vi "fotoncounter+lockin+fastratio_LV2010 GF VARIANT.vi"() -> ()   [LabVIEW 2014]
uses:
  Instance          14 40Saved   fotoncounter+lockin+fastratio v1 .vi
  Instance          13 40Saved   fotoncounter+lockin+fastratio v1 .vi
  Instance          33 40Saved   fotoncounter+lockin+fastratio v1 .vi
  Instance           2 40Saved   fotoncounter+lockin+fastratio v1 .vi
  Instance           5 40Saved   fotoncounter+lockin+fastratio v1 .vi
  Instance           6 40Saved   fotoncounter+lockin+fastratio v1 .vi
  Instance           7 40Saved   fotoncounter+lockin+fastratio v1 .vi
  Instance          15 40Saved   fotoncounter+lockin+fastratio v1 .vi
  Instance           8 40Saved   fotoncounter+lockin+fastratio v1 .vi
  Instance           9 40Saved   fotoncounter+lockin+fastratio v1 .vi
  Instance          10 40Saved   fotoncounter+lockin+fastratio v1 .vi
  Instance          11 40Saved   fotoncounter+lockin+fastratio v1 .vi
  Instance           1 40Saved   fotoncounter+lockin+fastratio v1 .vi
  Instance          18 40Saved   fotoncounter+lockin+fastratio v1 .vi
  Instance          19 40Saved   fotoncounter+lockin+fastratio v1 .vi
  Instance          23 40Saved   fotoncounter+lockin+fastratio v1 .vi
  Instance          17 40Saved   fotoncounter+lockin+fastratio v1 .vi
  Instance          22 40Saved   fotoncounter+lockin+fastratio v1 .vi
  Instance          20 40Saved   fotoncounter+lockin+fastratio v1 .vi
  Instance          21 40Saved   fotoncounter+lockin+fastratio v1 .vi
  Instance          26 40Saved   fotoncounter+lockin+fastratio v1 .vi
  Instance          27 40Saved   fotoncounter+lockin+fastratio v1 .vi
  Instance          29 40Saved   fotoncounter+lockin+fastratio v1 .vi
  <vilib>/Utility/file.llb/Write To Spreadsheet File (DBL).vi
  Instance          24 40Saved   fotoncounter+lockin+fastratio v1 .vi
  <vilib>/Utility/file.llb/Read From Spreadsheet File (DBL).vi
  Instance          32 40Saved   fotoncounter+lockin+fastratio v1 .vi
  Instance          31 40Saved   fotoncounter+lockin+fastratio v1 .vi
  Instance          30 40Saved   fotoncounter+lockin+fastratio v1 .vi
panel:
  in  "error in (no error)":errorcluster
  out "error out":errorcluster
  in  "Cluster":T1={"slope"=1, "Input Mode"=0, "time constant"=0, "display type"=0, "Range"=6} {"Range" items=["100 nV", "300 nV", "1 uV", "3 uV", "10 uV", "30 uV", "100 uV", "300 uV", "1 mV", "3 mV", "10 mV", "30 mV", "100 mV", "300 mV", "1 V", "3 V"]; "display type" items=["Output %", "Output calibrated ", "Ratio", "log Ratio", "ADC 1", "ADC 2", " ADC 3", "ADC 4", "Noise %", "Noise Calibrated", "Ref. Frequency"]; "time constant" items=["1 ms", "3 ms", "10 ms", "30 ms", "100 ms", "300 ms", "1 s", "3 s", "10 s", "30 s", "100 s", "300 s", "1 ks", "3 ks"]; "Input Mode" items=["Voltage Input ( A or A-B)", "Current Input 10E6 V/A", "Current Input 10E8 V/A"]; "slope" items=["6dB/octave", "12dB/octave"]}
  out "lockin":i32
  out "counter B":i32=147
  out "counter A":i32=5821
  out "LOCKIN OUTPUT DATA":cluster{"Y":dbl[], "Y":dbl[]}[](graph)=[{"Y"=[1.0], "Y"=[0.08234234]}]
  in  "EG&G 5209\nlockin amplifier\nGPIB address":u8=12 min=1 max=32 step=1
  out "# count periods done":i32=1
  out "Data Bit value":i32=1
  out "PHOTON COUNTER DATA":cluster{"all rows":dbl[], "all rows":dbl[]}[](graph)=[{"all rows"=[1.0], "all rows"=[5821.0]}, {"all rows"=[1.0], "all rows"=[147.0]}]
  in  "T select":i16(slide) scale=0.0..2.0
  in  "A scan step (V)":ext=-0.005 format="%.3e"
  in  "B scan step(V)":ext=-0.005 format="%.3e"
  in  "T scan step (V)":ext=0.02 format="%.3e"
  out "error 7":bool
  in  "A mode":bool=TRUE
  in  "B mode":bool=TRUE
  in  "T mode":bool=TRUE
  in  "A level (V)":ext=-0.025 format="%.3e"
  in  "B level (V)":ext=-0.025 format="%.3e"
  in  "T level (V)":ext=-0.01 format="%.3e"
  in  "B Preset":ext=1.0
  in  "count mode":i16(slide) scale=0.0..3.0 scale format="%.2f"
  in  "Path":path=path "C:/lvtemp/phototemp"
  out "error 6":bool
  in  "A slope":bool
  in  "B slope":bool
  in  "T slope":bool
  in  "trigger slope":bool
  out "error 5":bool
  in  "trigger level":ext=2.0 format="%.3f"
  in  "A scan step":ext=0.000005 format="%.3e"
  in  "dwell source":i32(slide) scale=0.0..1.0
  in  "dwell time":ext=0.1 format="%.4f"
  in  "# count periods\n(2000 max.)":i32=1
  in  "A select":i16(slide)=1 scale=0.0..1.0
  in  "B select":i16(slide)=1 scale=1.0..2.0 scale format="%.2f"
  in  "SR400\nphoton counter\nGPIB address":string="0:23"
  in  "B gate delay":ext=0.00027000000000000000001 format="%.3e"
  in  "B gate mode":i16(slide)=1 scale=0.0..2.0
  out "error 2":bool
  in  "B gate width":ext=0.00021 format="%.3e"
  in  "B scan step":ext=0.000005 format="%.3e"
  in  "A gate delay":ext=0.00001 format="%.3e"
  in  "A gate mode":i16(slide)=1 scale=0.0..2.0 scale format="%.2f"
  in  "A gate width":ext=0.00021 format="%.3e"
  in  "T Preset":ext=1.0
  # "SR400 PHOTON COUNTER + EG&G 5209 LOCKIN AMPLIFIER"
  # "ADDRESSING/TRIGGER/DWELL SETTINGS"
  # "COUNTER/INPUT SETTINGS"
  # "photon counter GPIB Board 0, address 23\nEG&G lockin GPIB Board 0, address 12"
  # "RISE\n\nFALL"
  # "(s)"
  # "note: valid dwell time\n0.002  to 60.0 s"
  # "(s)"
  # "DISCRIMINATOR SETTINGS"
  # "GATE SETTINGS"
  # "FIXED\n\nSCAN"
  # "RISE\n\nFALL"
  # "RISE\n\nFALL"
  # "FIXED\n\nSCAN"
  # "FIXED\n\nSCAN"
  # "RISE\n\nFALL"
  # "note: valid disc levels \n-0.30 to 0.30 V"
  # "note: valid scan steps \n-0.020 to 0.020 V"
  # "\"...The greatest trick the Devil ever pulled was convincing the world he didn't exist...\" (and then inventing LabView)..."
  # "This makes the lockin work again. no idea if the settings are right, or even need to be messed with"
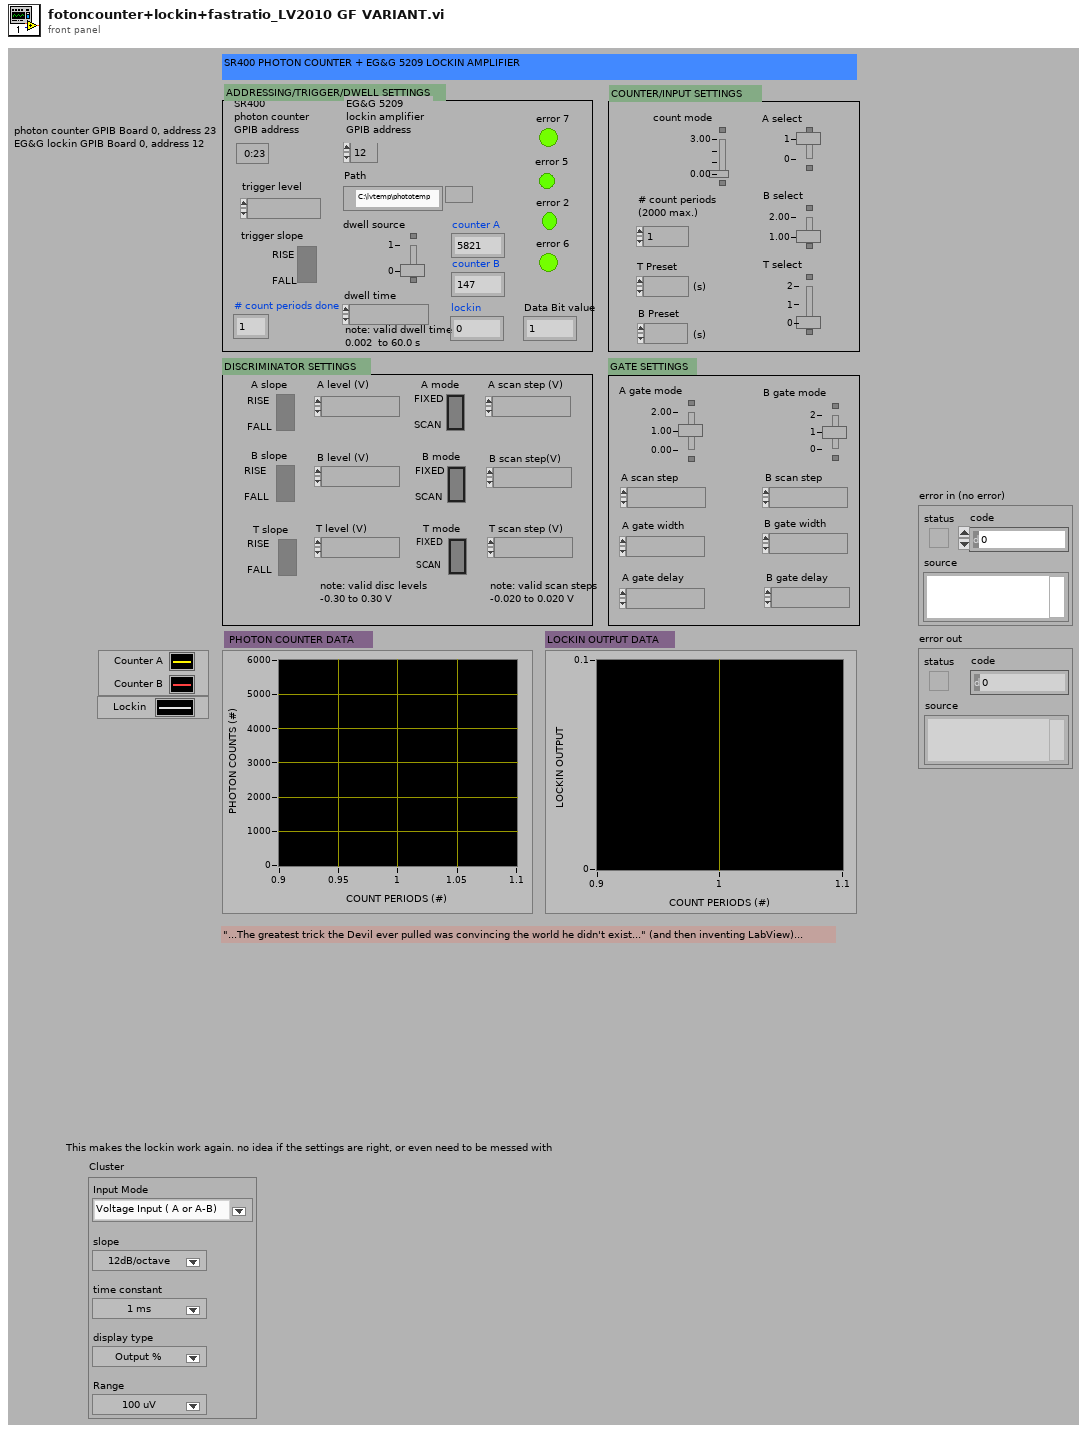
[diagram p1: front panel]
types:
  T1 = cluster{"slope":i32, "Input Mode":i32, "time constant":i32, "display type":i32, "Range":i32}
  T2 = enum16{"open", "open or create", "create or replace", "create", "open (read only)"}
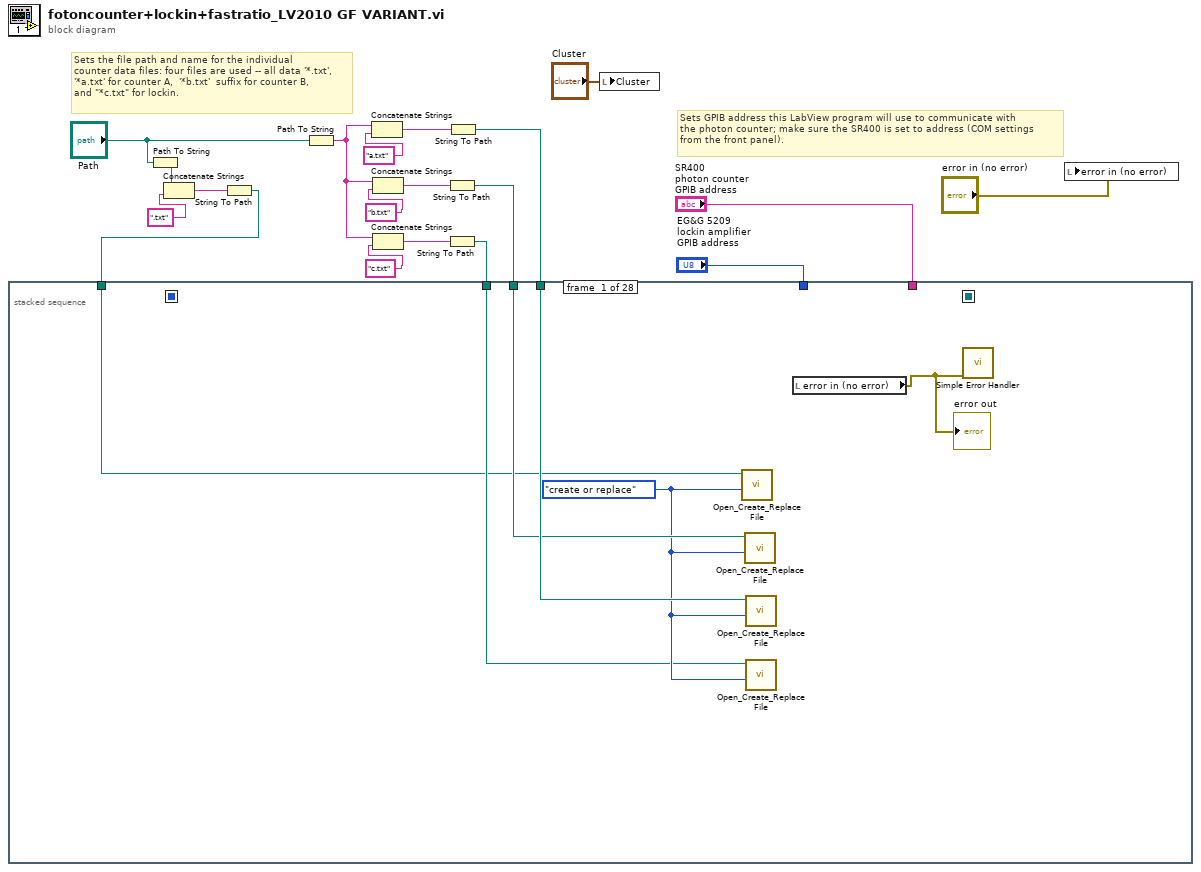
[diagram p0: block diagram]
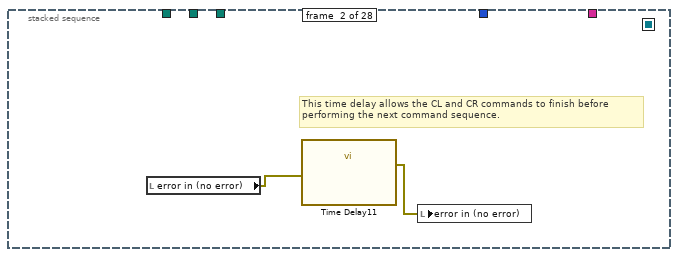
[diagram p2: hidden frame]
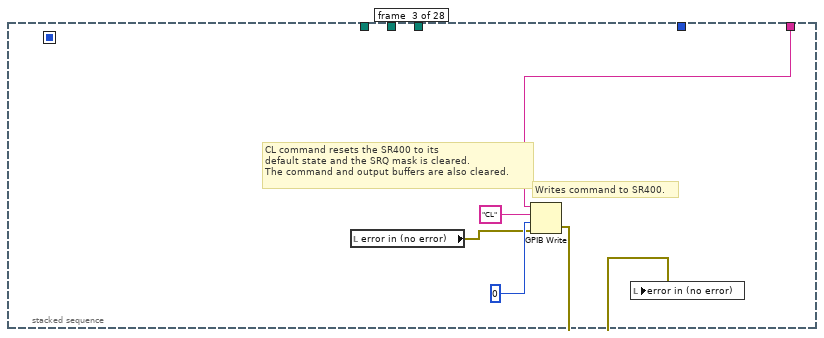
[diagram p3: hidden frame]
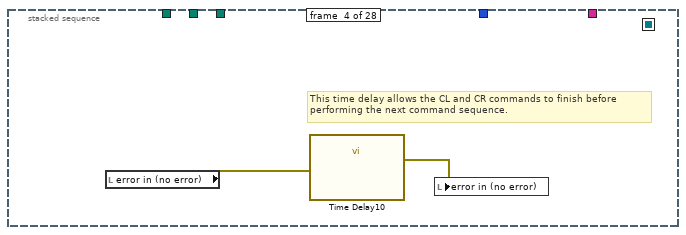
[diagram p4: hidden frame]
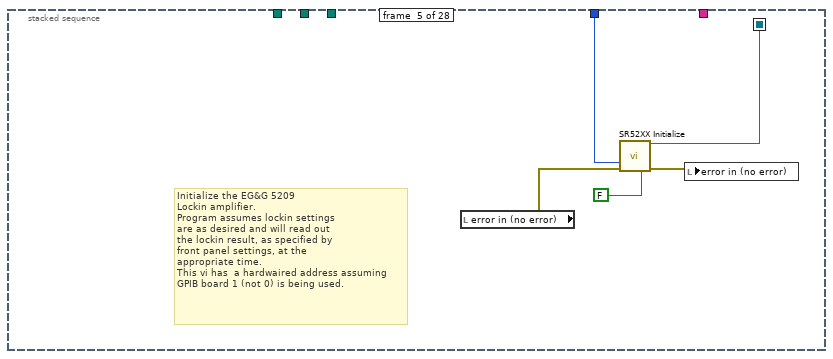
[diagram p5: hidden frame]
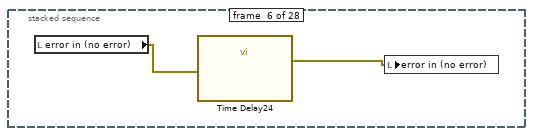
[diagram p6: hidden frame]
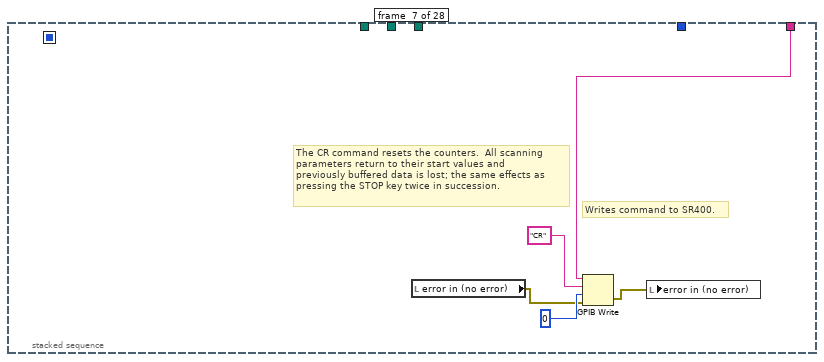
[diagram p7: hidden frame]
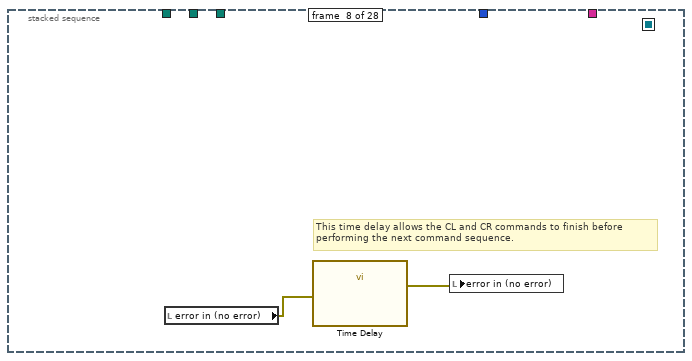
[diagram p8: hidden frame]
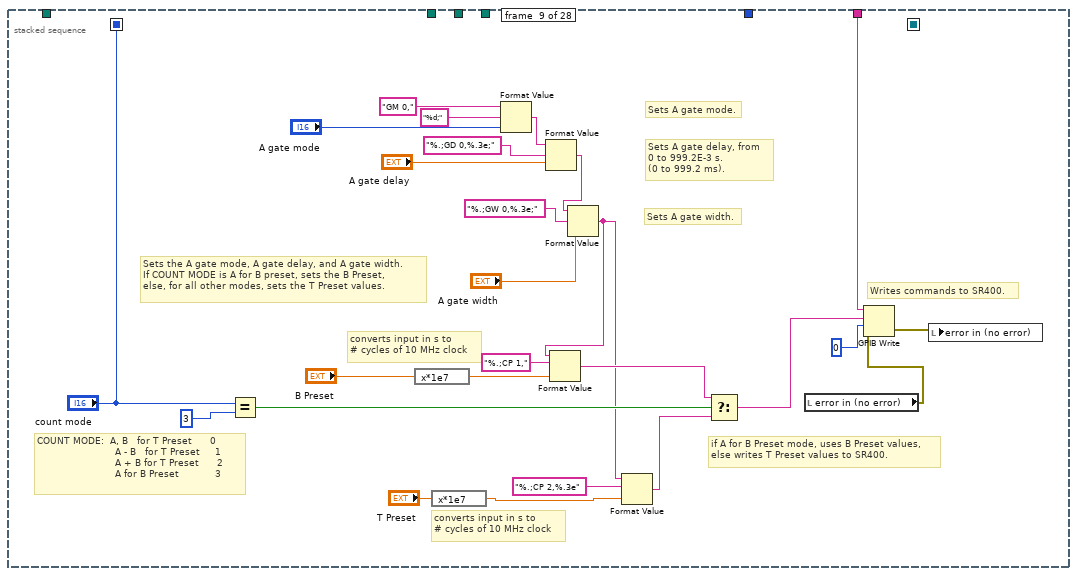
[diagram p9: hidden frame]
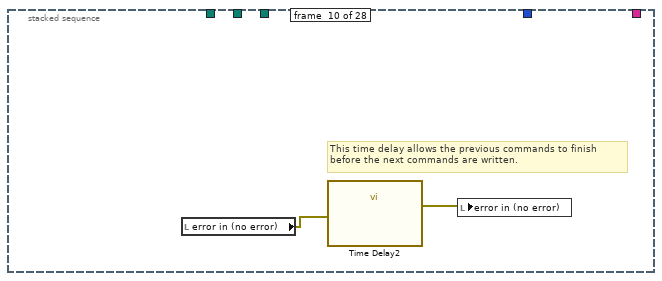
[diagram p10: hidden frame]
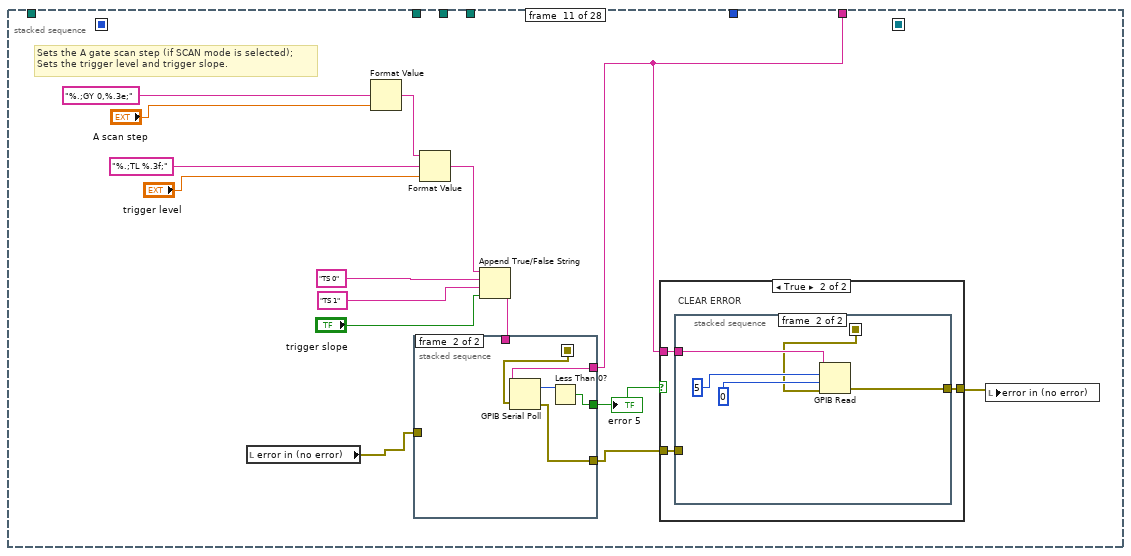
[diagram p11: hidden frame]
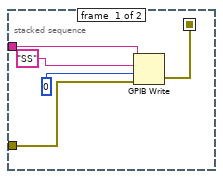
[diagram p13: hidden frame]
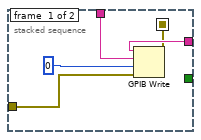
[diagram p14: hidden frame]
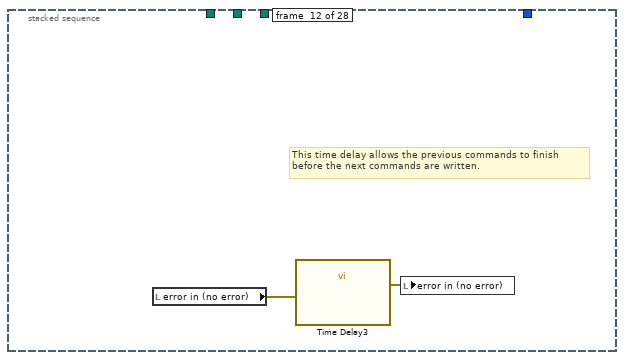
[diagram p15: hidden frame]
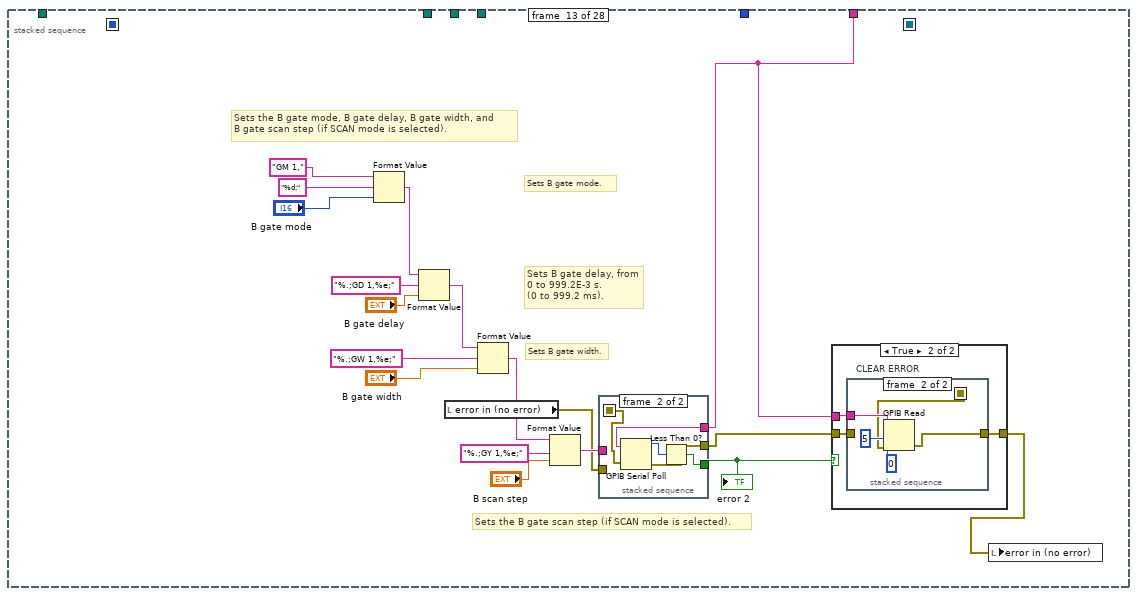
[diagram p16: hidden frame]
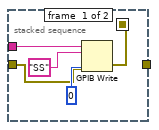
[diagram p18: hidden frame]
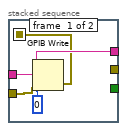
[diagram p19: hidden frame]
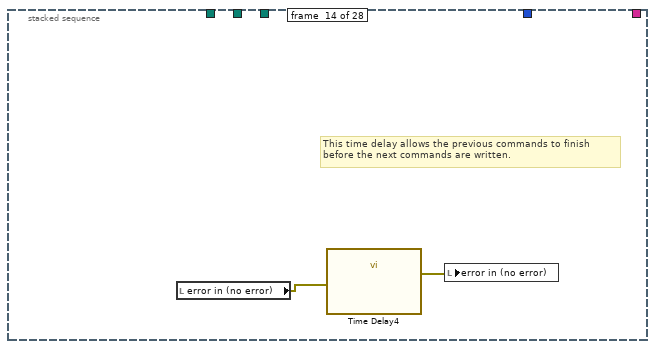
[diagram p20: hidden frame]
diagram:
  # "Sets the file path and name for the individual\ncounter data files: four files are used -- all data '*.txt',\n'*a.txt' for counter A,  '*b.txt'  suffix for counter B,\nand \"*c.txt\" for lockin."
  # "Sets GPIB address this LabView program will use to communicate with\nthe photon counter; make sure the SR400 is set to address (COM settings\nfrom the front panel)."
  n1 = Path To String(path="Path") -> (string=w13:string)
  n2 = Concatenate Strings(w13, ".txt") -> (w11:string)
  n3 = String To Path(string=w11) -> (path=w3:path)
  n4 = Path To String(path="Path") -> (string=w6:string)
  n5 = Concatenate Strings(w6, "a.txt") -> (w14:string)
  n6 = Concatenate Strings(w6, "b.txt") -> (w17:string)
  n7 = Concatenate Strings(w6, "c.txt") -> (w8:string)
  n8 = String To Path(string=w17) -> (path=w15:path)
  n9 = String To Path(string=w8) -> (path=w5:path)
  n10 = String To Path(string=w14) -> (path=w16:path)
  n11 = stacked-sequence {
    seq-local: [_ _ _ _ _ _ _ _ "count mode" _ _ _ _ _ _ _ _ _ _ _ _ _ _ _ _ _ _ _] -> [_ _ _ _ _ _ _ _ _ _ _ _ _ _ _ _ _ _ _ _ _ _ _ _ _ _ w274 _]
    seq-local: [_ _ _ _ w37 _ _ _ _ _ _ _ _ _ _ _ _ _ _ _ _ _ _ _ _ _ _ _] -> [_ _ _ _ _ _ _ _ _ _ _ _ _ _ _ _ _ _ _ _ _ _ _ _ _ _ w273 _]
    tunnel: "SR400\nphoton counter\nGPIB address" -> [_ _ w30 _ _ _ w44 _ w69 _ w80 _ w122 _ w166 _ w179 _ w189 _ w203 _ w231 _ w259 _ w280 _]
    tunnel: w16 -> [w25 _ _ _ _ _ _ _ _ _ _ _ _ _ _ _ _ _ _ _ _ _ _ _ _ _ w279 _]
    tunnel: w15 -> [w24 _ _ _ _ _ _ _ _ _ _ _ _ _ _ _ _ _ _ _ _ _ _ _ _ _ w278 _]
    tunnel: w3 -> [w21 _ _ _ _ _ _ _ _ _ _ _ _ _ _ _ _ _ _ _ _ _ _ _ _ _ w277 w469]
    tunnel: "EG&G 5209\nlockin amplifier\nGPIB address" -> [_ _ _ _ w38 _ _ _ _ _ _ _ _ _ _ _ _ _ _ _ _ _ _ _ _ _ _ _]
    tunnel: w5 -> [w22 _ _ _ _ _ _ _ _ _ _ _ _ _ _ _ _ _ _ _ _ _ _ _ _ _ w276 _]
    frame #0 {
      w23 = T2."create or replace" ("function (open:0)")
      n12 = call <vilib>:"Open_Create_Replace File.vi"("function (open:0)"=w23, "file path"=w21) -> ()  [unwired: 6 in, 4 out]
      n13 = call <vilib>:"Open_Create_Replace File.vi"("function (open:0)"=w23, "file path"=w24) -> ()  [unwired: 6 in, 4 out]
      n14 = call <vilib>:"Open_Create_Replace File.vi"("function (open:0)"=w23, "file path"=w25) -> ()  [unwired: 6 in, 4 out]
      n15 = call <vilib>:"Open_Create_Replace File.vi"("function (open:0)"=w23, "file path"=w22) -> ()  [unwired: 6 in, 4 out]
      n16 = local read "error in (no error)"() -> (w20:errorcluster)
      "error out" <- w20
      n17 = call <vilib>:"Simple Error Handler.vi"("error in (no error)"=w20) -> ()  [unwired: 4 in, 5 out]
    }
    frame #1 {
      # "This time delay allows the CL and CR commands to finish before\nperforming the next command sequence."
      n18 = local read "error in (no error)"() -> (w27:errorcluster)
      n19 = call "Time Delay11"("error in (no error)"=w27) -> ("error out"=w26:errorcluster)  [unwired: 10 in]
      n20 = local write "error in (no error)"(w26) -> ()
    }
    frame #2 {
      # "Writes command to SR400."
      # "CL command resets the SR400 to its\ndefault state and the SRQ mask is cleared.\nThe command and output buffers are also cleared."
      n21 = local read "error in (no error)"() -> (w29:errorcluster)
      n22 = GPIB Write(0:w30, 1:"CL", 2:0, 3:w29) -> (6:w28:errorcluster)  [unwired: 1 in, 1 out]
      n23 = local write "error in (no error)"(w28) -> ()
    }
    frame #3 {
      # "This time delay allows the CL and CR commands to finish before\nperforming the next command sequence."
      n24 = local read "error in (no error)"() -> (w33:errorcluster)
      n25 = call "Time Delay10"("error in (no error)"=w33) -> ("error out"=w34:errorcluster)  [unwired: 10 in]
      n26 = local write "error in (no error)"(w34) -> ()
    }
    frame #4 {
      # "Initialize the EG&G 5209\nLockin amplifier.\nProgram assumes lockin settings\nare as desired and will read out\nthe lockin result, as specified by \nfront panel settings, at the\nappropriate time.\nThis vi has  a hardwaired address assuming \nGPIB board 1 (not 0) is being used."
      n27 = local read "error in (no error)"() -> (w35:errorcluster)
      n28 = call "SR52XX Initialize.vi"("Port"=w38, "error in (no error)"=w35, "reset"=FALSE) -> ("VISA session"=w37:refnum<visa-resource-name>, "error out"=w36:errorcluster)  [unwired: 10 in, 1 out]
      n29 = local write "error in (no error)"(w36) -> ()
    }
    frame #5 {
      n30 = local read "error in (no error)"() -> (w40:errorcluster)
      n31 = call "Time Delay24"("error in (no error)"=w40) -> ("error out"=w41:errorcluster)  [unwired: 10 in]
      n32 = local write "error in (no error)"(w41) -> ()
    }
    frame #6 {
      # "Writes command to SR400."
      # "The CR command resets the counters.  All scanning\nparameters return to their start values and \npreviously buffered data is lost; the same effects as\npressing the STOP key twice in succession."
      n33 = local read "error in (no error)"() -> (w42:errorcluster)
      n34 = GPIB Write(0:w44, 1:"CR", 2:0, 3:w42) -> (6:w43:errorcluster)  [unwired: 1 in, 1 out]
      n35 = local write "error in (no error)"(w43) -> ()
    }
    frame #7 {
      # "This time delay allows the CL and CR commands to finish before\nperforming the next command sequence."
      n36 = local read "error in (no error)"() -> (w48:errorcluster)
      n37 = call "Time Delay"("error in (no error)"=w48) -> ("error out"=w47:errorcluster)  [unwired: 10 in]
      n38 = local write "error in (no error)"(w47) -> ()
    }
    frame #8 {
      # "if A for B Preset mode, uses B Preset values,\nelse writes T Preset values to SR400."
      # "converts input in s to\n# cycles of 10 MHz clock"
      # "converts input in s to\n# cycles of 10 MHz clock"
      # "Writes commands to SR400."
      # "Sets A gate delay, from \n0 to 999.2E-3 s.\n(0 to 999.2 ms)."
      # "Sets A gate width."
      # "Sets A gate mode."
      # "COUNT MODE:  A, B   for T Preset      0 \n                          A - B   for T Preset     1\n                          A + B for T Preset      2\n                          A for B Preset            3"
      # "Sets the A gate mode, A gate delay, and A gate width.\nIf COUNT MODE is A for B preset, sets the B Preset, \nelse, for all other modes, sets the T Preset values."
      n39 = Equal?(x="count mode", y=3) -> (x = y?=w61:bool)
      n40 = expression code="x*1e7"("B Preset") -> (w51:ext)
      n41 = expression code="x*1e7"("T Preset") -> (w53:ext)
      n42 = Format Value(string ("")="GM 0,", format string="%d;", value (0)="A gate mode") -> (output string=w68:string)
      n43 = Format Value(string ("")=w68, format string="%.;GD 0,%.3e;", value (0)="A gate delay") -> (output string=w65:string)
      n44 = Format Value(string ("")=w65, format string="%.;GW 0,%.3e;", value (0)="A gate width") -> (output string=w56:string)
      n45 = Format Value(string ("")=w56, format string="%.;CP 1,", value (0)=w51) -> (output string=w57:string)
      n46 = Format Value(string ("")=w56, format string="%.;CP 2,%.3e", value (0)=w53) -> (output string=w59:string)
      n47 = Select(t=w57, s=w61, f=w59) -> (s? t:f=w55:string)
      n48 = local read "error in (no error)"() -> (w49:errorcluster)
      n49 = GPIB Write(0:w69, 1:w55, 2:0, 3:w49) -> (6:w50:errorcluster)  [unwired: 1 in, 1 out]
      n50 = local write "error in (no error)"(w50) -> ()
    }
    frame #9 {
      # "This time delay allows the previous commands to finish \nbefore the next commands are written."
      n51 = local read "error in (no error)"() -> (w76:errorcluster)
      n52 = call "Time Delay2"("error in (no error)"=w76) -> ("error out"=w75:errorcluster)  [unwired: 10 in]
      n53 = local write "error in (no error)"(w75) -> ()
    }
    frame #10 {
      # "Sets the A gate scan step (if SCAN mode is selected); \nSets the trigger level and trigger slope."
      n54 = local read "error in (no error)"() -> (w79:errorcluster)
      n55 = Format Value(format string="%.;GY 0,%.3e;", value (0)="A scan step") -> (output string=w84:string)  [unwired: 1 in]
      n56 = Format Value(string ("")=w84, format string="%.;TL %.3f;", value (0)="trigger level") -> (output string=w87:string)
      n57 = Append True/False String(1:"trigger slope", 2:"TS 1", 3:"TS 0", 4:w87) -> (0:w91:string)
      n58 = stacked-sequence {
        seq-local: [w106 _] -> [_ w112]
        tunnel: w80 -> [w109 w113]
        tunnel: w91 -> [w108 _]
        tunnel: [_ w115] -> w82
        tunnel: w79 -> [w107 _]
        tunnel: [_ w111] -> w78
        frame #0 {
          n59 = GPIB Write(0:w109, 1:w108, 2:0, 3:w107) -> (6:w106:errorcluster)  [unwired: 1 in, 1 out]
        }
        frame #1 {
          n60 = GPIB Serial Poll(0:w113, 1:w112) -> (2:w114:i16, 4:w111:errorcluster)  [unwired: 1 out]
          n61 = Less Than 0?(x=w114) -> (x < 0?=w115:bool)
        }
      }
      "error 5" <- w82
      n62 = case shown="True" w82 {
        tunnel: w80 -> [_ w95]
        tunnel: w78 -> [w92 w94]
        tunnel: [w92 w93] -> w77
        frame False {
          # "NO ERROR."
        }
        frame True {
          # "CLEAR ERROR"
          n63 = stacked-sequence {
            seq-local: [w96 _] -> [_ w102]
            tunnel: w95 -> [w98 w103]
            tunnel: w94 -> [w97 _]
            tunnel: [_ w101] -> w93
            frame #0 {
              n64 = GPIB Write(0:w98, 1:"SS", 2:0, 3:w97) -> (6:w96:errorcluster)  [unwired: 1 in, 1 out]
            }
            frame #1 {
              n65 = GPIB Read(0:w103, 1:5, 2:0, 3:w102) -> (7:w101:errorcluster)  [unwired: 1 in, 2 out]
            }
          }
        }
      }
      n66 = local write "error in (no error)"(w77) -> ()
    }
    frame #11 {
      # "This time delay allows the previous commands to finish \nbefore the next commands are written."
      n67 = local read "error in (no error)"() -> (w117:errorcluster)
      n68 = call "Time Delay3"("error in (no error)"=w117) -> ("error out"=w116:errorcluster)  [unwired: 10 in]
      n69 = local write "error in (no error)"(w116) -> ()
    }
    frame #12 {
      # "Sets the B gate scan step (if SCAN mode is selected)."
      # "Sets B gate width."
      # "Sets B gate delay, from \n0 to 999.2E-3 s.\n(0 to 999.2 ms)."
      # "Sets B gate mode."
      # "Sets the B gate mode, B gate delay, B gate width, and \nB gate scan step (if SCAN mode is selected)."
      n70 = Format Value(string ("")="GM 1,", format string="%d;", value (0)="B gate mode") -> (output string=w127:string)
      n71 = Format Value(string ("")=w127, format string="%.;GD 1,%e;", value (0)="B gate delay") -> (output string=w121:string)
      n72 = local read "error in (no error)"() -> (w120:errorcluster)
      n73 = Format Value(string ("")=w121, format string="%.;GW 1,%e;", value (0)="B gate width") -> (output string=w131:string)
      n74 = Format Value(string ("")=w131, format string="%.;GY 1,%e;", value (0)="B scan step") -> (output string=w134:string)
      n75 = stacked-sequence {
        seq-local: [w150 _] -> [_ w156]
        tunnel: w122 -> [w152 w157]
        tunnel: [_ w159] -> w135
        tunnel: w134 -> [w154 _]
        tunnel: w120 -> [w151 _]
        tunnel: [_ w155] -> w119
        frame #0 {
          n76 = GPIB Write(0:w152, 1:w154, 2:0, 3:w151) -> (6:w150:errorcluster)  [unwired: 1 in, 1 out]
        }
        frame #1 {
          n77 = GPIB Serial Poll(0:w157, 1:w156) -> (2:w158:i16, 4:w155:errorcluster)  [unwired: 1 out]
          n78 = Less Than 0?(x=w158) -> (x < 0?=w159:bool)
        }
      }
      "error 2" <- w135
      n79 = case shown="True" w135 {
        tunnel: w122 -> [_ w139]
        tunnel: w119 -> [w136 w138]
        tunnel: [w136 w137] -> w118
        frame False {
          # "NO ERROR."
        }
        frame True {
          # "CLEAR ERROR"
          n80 = stacked-sequence {
            seq-local: [w140 _] -> [_ w146]
            tunnel: w139 -> [w142 w147]
            tunnel: w138 -> [w141 _]
            tunnel: [_ w145] -> w137
            frame #0 {
              n81 = GPIB Write(0:w142, 1:"SS", 2:0, 3:w141) -> (6:w140:errorcluster)  [unwired: 1 in, 1 out]
            }
            frame #1 {
              n82 = GPIB Read(0:w147, 1:5, 2:0, 3:w146) -> (7:w145:errorcluster)  [unwired: 1 in, 2 out]
            }
          }
        }
      }
      n83 = local write "error in (no error)"(w118) -> ()
    }
    frame #13 {
      # "This time delay allows the previous commands to finish \nbefore the next commands are written."
      n84 = local read "error in (no error)"() -> (w161:errorcluster)
      n85 = call "Time Delay4"("error in (no error)"=w161) -> ("error out"=w160:errorcluster)  [unwired: 10 in]
      n86 = local write "error in (no error)"(w160) -> ()
    }
    frame #14 {
      # "Writes commands to SR400."
      # "Sets the input to counter A (INPUT1 or 10 MHz clock);\nSets the input to counter B (INPUT1 or INPUT2);"
      n87 = Format Value(string ("")="CI 0,", format string="%d;", value (0)="A select") -> (output string=w171:string)
      n88 = Format Value(string ("")=w171, format string="%.;CI 1,%d;", value (0)="B select") -> (output string=w164:string)
      n89 = local read "error in (no error)"() -> (w163:errorcluster)
      n90 = GPIB Write(0:w166, 1:w164, 2:0, 3:w163) -> (6:w162:errorcluster)  [unwired: 1 in, 1 out]
      n91 = local write "error in (no error)"(w162) -> ()
    }
    frame #15 {
      # "This time delay allows the previous commands to finish \nbefore the next commands are written."
      n92 = local read "error in (no error)"() -> (w174:errorcluster)
      n93 = call "Time Delay12"("error in (no error)"=w174) -> ("error out"=w173:errorcluster)  [unwired: 10 in]
      n94 = local write "error in (no error)"(w173) -> ()
    }
    frame #16 {
      # "Writes commands to SR400."
      # "Sets the input to counter T (EXT TRIG, INPUT 2, or 10 MHz clock);"
      n95 = local read "error in (no error)"() -> (w176:errorcluster)
      n96 = Pick Line(string ("")="CI 2,", multi-line string="0;\r2;\r3;", line index="T select") -> (output string=w178:string)
      n97 = GPIB Write(0:w179, 1:w178, 2:0, 3:w176) -> (6:w175:errorcluster)  [unwired: 1 in, 1 out]
      n98 = local write "error in (no error)"(w175) -> ()
    }
    frame #17 {
      # "This time delay allows the previous commands to finish \nbefore the next commands are written."
      n99 = local read "error in (no error)"() -> (w184:errorcluster)
      n100 = call "Time Delay5"("error in (no error)"=w184) -> ("error out"=w183:errorcluster)  [unwired: 10 in]
      n101 = local write "error in (no error)"(w183) -> ()
    }
    frame #18 {
      # "Writes commands to SR400."
      # "B counter discriminator level"
      # "T counter discriminator level"
      # "A counter discriminator level"
      # "Sets the A, B, and T discriminator levels.  \nThe input values must be between \n-0.3 V and 0.3 V (-300 mV and 300 mV)\nor else the counter leaves the default values\nof -0.01 V (-10 mV)."
      n102 = Format Value(string ("")="DL 0,", format string="%.4e;DL 1,", value (0)="A level (V)") -> (output string=w193:string)
      n103 = Format Value(string ("")=w193, format string="%.4e;DL 2,", value (0)="B level (V)") -> (output string=w194:string)
      n104 = Format Value(string ("")=w194, format string="%.4e;", value (0)="T level (V)") -> (output string=w187:string)
      n105 = local read "error in (no error)"() -> (w186:errorcluster)
      n106 = GPIB Write(0:w189, 1:w187, 2:0, 3:w186) -> (6:w185:errorcluster)  [unwired: 1 in, 1 out]
      n107 = local write "error in (no error)"(w185) -> ()
    }
    frame #19 {
      # "This time delay allows the previous commands to finish \nbefore the next commands are written."
      n108 = local read "error in (no error)"() -> (w200:errorcluster)
      n109 = call "Time Delay7"("error in (no error)"=w200) -> ("error out"=w199:errorcluster)  [unwired: 10 in]
      n110 = local write "error in (no error)"(w199) -> ()
    }
    frame #20 {
      # "Sets the slope of the A, B, and T\ndiscriminator levels  (rise or fall)."
      n111 = local read "error in (no error)"() -> (w202:errorcluster)
      n112 = Append True/False String(1:"A slope", 2:"DS 0,1;", 3:"DS 0,0;") -> (0:w210:string)  [unwired: 1 in]
      n113 = Append True/False String(1:"B slope", 2:"DS 1,1;", 3:"DS 1,0;", 4:w210) -> (0:w213:string)
      n114 = Append True/False String(1:"T slope", 2:"DS 2,1;", 3:"DS 2,0;", 4:w213) -> (0:w216:string)
      n115 = stacked-sequence {
        seq-local: [w217 _] -> [_ w223]
        tunnel: w203 -> [w220 w226]
        tunnel: w216 -> [w221 _]
        tunnel: [_ w224] -> w206
        tunnel: w202 -> [w218 _]
        tunnel: [_ w222] -> w201
        frame #0 {
          n116 = GPIB Write(0:w220, 1:w221, 2:0, 3:w218) -> (6:w217:errorcluster)  [unwired: 1 in, 1 out]
        }
        frame #1 {
          n117 = GPIB Serial Poll(0:w226, 1:w223) -> (2:w225:i16, 4:w222:errorcluster)  [unwired: 1 out]
          n118 = Less Than 0?(x=w225) -> (x < 0?=w224:bool)
        }
      }
      "error 6" <- w206
      n119 = local write "error in (no error)"(w201) -> ()
    }
    frame #21 {
      # "This time delay allows the previous commands to finish \nbefore the next commands are written."
      n120 = local read "error in (no error)"() -> (w228:errorcluster)
      n121 = call "Time Delay8"("error in (no error)"=w228) -> ("error out"=w227:errorcluster)  [unwired: 10 in]
      n122 = local write "error in (no error)"(w227) -> ()
    }
    frame #22 {
      # "Sets the mode of the A, B, and T\ndiscriminators  (FIXED or SCAN)."
      n123 = local read "error in (no error)"() -> (w230:errorcluster)
      n124 = Append True/False String(1:"A mode", 2:"DM 0,1;", 3:"DM 0,0;") -> (0:w238:string)  [unwired: 1 in]
      n125 = Append True/False String(1:"B mode", 2:"DM 1,1;", 3:"DM 1,0;", 4:w238) -> (0:w241:string)
      n126 = Append True/False String(1:"T mode", 2:"DM 2,1;", 3:"DM 2,0;", 4:w241) -> (0:w244:string)
      n127 = stacked-sequence {
        seq-local: [w245 _] -> [_ w251]
        tunnel: w231 -> [w248 w254]
        tunnel: w244 -> [w249 _]
        tunnel: [_ w252] -> w234
        tunnel: w230 -> [w246 _]
        tunnel: [_ w250] -> w229
        frame #0 {
          n128 = GPIB Write(0:w248, 1:w249, 2:0, 3:w246) -> (6:w245:errorcluster)  [unwired: 1 in, 1 out]
        }
        frame #1 {
          n129 = GPIB Serial Poll(0:w254, 1:w251) -> (2:w253:i16, 4:w250:errorcluster)  [unwired: 1 out]
          n130 = Less Than 0?(x=w253) -> (x < 0?=w252:bool)
        }
      }
      "error 7" <- w234
      n131 = local write "error in (no error)"(w229) -> ()
    }
    frame #23 {
      # "This time delay allows the previous commands to finish \nbefore the next commands are written."
      n132 = local read "error in (no error)"() -> (w256:errorcluster)
      n133 = call "Time Delay9"("error in (no error)"=w256) -> ("error out"=w255:errorcluster)  [unwired: 10 in]
      n134 = local write "error in (no error)"(w255) -> ()
    }
    frame #24 {
      # "Writes commands to SR400."
      # "B  discriminator scan step"
      # "T  discriminator scan step"
      # "A discriminator scan step"
      # "Sets the A, B, and T discriminator \nscan step size.  The input values must be between \n-0.02 V and 0.02 V (-20 mV and 20 mV)."
      n135 = Format Value(string ("")="DY 0,", format string="%.4e;DY 1,", value (0)="A scan step (V)") -> (output string=w265:string)
      n136 = Format Value(string ("")=w265, format string="%.4e;DY 2,", value (0)="B scan step(V)") -> (output string=w266:string)
      n137 = Format Value(string ("")=w266, format string="%.4e;", value (0)="T scan step (V)") -> (output string=w260:string)
      n138 = local read "error in (no error)"() -> (w258:errorcluster)
      n139 = GPIB Write(0:w259, 1:w260, 2:0, 3:w258) -> (6:w257:errorcluster)  [unwired: 1 in, 1 out]
      n140 = local write "error in (no error)"(w257) -> ()
    }
    frame #25 {
      # "This time delay allows the previous commands to finish \nbefore triggering the scan, taking the data, and reading\nout the buffer.."
      n141 = local read "error in (no error)"() -> (w272:errorcluster)
      n142 = call "Time Delay6"("error in (no error)"=w272) -> ("error out"=w271:errorcluster)  [unwired: 10 in]
      n143 = local write "error in (no error)"(w271) -> ()
    }
    frame #26 {
      # "Path describes filename and location for\nwavelength, counter A, and counter B data\nto be written; also writesadditional files\nwith wavelength, counter A ('a'  suffix) and\nwith wavelgnth, counter B data ('b' suffix)."
      n144 = stacked-sequence {
        tunnel: "# count periods\n(2000 max.)" -> [w287 _ w309 _ _]
        tunnel: w274 -> [w294 _ w305 _ _]
        tunnel: w280 -> [w285 w302 w306 w460 w465]
        tunnel: w279 -> [_ _ w310 _ _]
        tunnel: w278 -> [_ _ w307 _ _]
        tunnel: w277 -> [_ _ w308 _ _]
        tunnel: w273 -> [_ _ w303 _ _]
        tunnel: w276 -> [_ _ w304 _ _]
        frame #0 {
          # "COUNT RESET (CR); \nSRQ AT END OF SCAN (SV 4); \n# PERIODS (NP);\n COUNT MODE: A,B FOR T (CM 0), \n                          A-B for T (CM 1), \n                          A+B for T (CM 2), \n                          A FOR B (CM 3);\nSet DWELL SOURCE and DWELL TIME;"
          # "Resets the counters; sets the count periods,\nthe count mode, dwell source and dwell time."
          n145 = Format Value(string ("")="CR;SV 4;", format string="NP %d;", value (0)=w287) -> (output string=w293:string)
          n146 = Pick Line(string ("")=w293, multi-line string="CM 0;\nCM 1;\n\rCM 2;\rCM 3;", line index=w294) -> (output string=w283:string)
          n147 = case shown="..0" "dwell source" {
            tunnel: ["dwell time" ext 0.0] -> w284
            frame ..0 {
            }
            frame 1.. {
              # "EXTERNAL"
            }
          }
          n148 = local read "error in (no error)"() -> (w282:errorcluster)
          n149 = Format Value(string ("")=w283, format string="%.;DT %f", value (0)=w284) -> (output string=w291:string)
          n150 = GPIB Write(0:w285, 1:w291, 2:3, 3:w282) -> (6:w281:errorcluster)  [unwired: 1 in, 1 out]
          n151 = local write "error in (no error)"(w281) -> ()
        }
        frame #1 {
          # "Starts a new scan."
          n152 = local read "error in (no error)"() -> (w299:errorcluster)
          n153 = GPIB Write(0:w302, 1:"CS", 2:3, 3:w299) -> (6:w298:errorcluster)  [unwired: 1 in, 1 out]
          n154 = local write "error in (no error)"(w298) -> ()
        }
        frame #2 {
          n155 = for {
            N: w309 -> [_]
            tunnel: w306 -> [w313]
            tunnel: w310 -> [w316]
            tunnel: w308 -> [w317]
            tunnel: w307 -> [w315]
            tunnel: w305 -> [w314]
            tunnel: w303 -> [w312]
            tunnel: w304 -> [w311]
            n156 = stacked-sequence {
              seq-local: [_ _ _ w347 _ _ _ _ _ _ _ _ _ _ _ _ _ _ _ _ _] -> [_ _ _ _ _ _ _ w366 _ _ _ w389 _ _ _ w413 _ w424 _ _ _]
              seq-local: [_ _ _ _ _ _ _ w363 _ _ _ _ _ _ _ _ _ _ _ _ _] -> [_ _ _ _ _ _ _ _ _ _ _ _ _ _ _ _ _ w426 _ _ _]
              seq-local: [_ _ _ _ _ _ _ _ _ _ _ w386 _ _ _ _ _ _ _ _ _] -> [_ _ _ _ _ _ _ _ _ _ _ _ _ _ _ _ _ w423 _ _ _]
              seq-local: [_ _ _ _ _ _ _ _ _ _ _ _ _ w408 _ _ _ _ _ _ _] -> [_ _ _ _ _ _ _ _ _ _ _ _ _ _ _ w412 _ w422 _ _ _]
              tunnel: w317 -> [_ _ _ _ _ _ _ _ _ _ _ _ _ _ _ _ _ w421 _ _ _]
              tunnel: w316 -> [_ _ _ _ _ _ _ w365 _ _ _ _ _ _ _ _ _ _ _ w432 _]
              tunnel: w315 -> [_ _ _ _ _ _ _ _ _ _ _ w387 _ _ _ _ _ _ _ w445 _]
              tunnel: w314 -> [_ _ _ _ _ _ _ _ _ _ _ _ _ _ _ _ _ _ _ _ _]
              tunnel: w313 -> [w318 w340 _ w349 _ w356 _ w370 _ w379 _ w390 _ _ _ _ _ _ _ _ _]
              tunnel: w312 -> [_ _ _ _ _ _ _ _ _ _ _ _ _ w409 _ _ _ _ _ _ _]
              tunnel: w311 -> [_ _ _ _ _ _ _ _ _ _ _ _ _ _ _ w414 _ _ _ _ w448]
              frame #0 {
                n157 = while {
                  tunnel: w318 -> [w320]
                  stop <- w319 stop-if-true
                  n158 = stacked-sequence {
                    tunnel: w320 -> [w323 _ w333 _]
                    tunnel: [_ _ w331 _] -> w319
                    frame #0 {
                      # "SS command reads the status bit: Bit 1\nindicates DATA READY, set at the end \nof each count period to indicate that counter\ndata is available."
                      # "Writes command to SR400;\nRead the status byte, bit 1;\nData Ready."
                      n159 = local read "error in (no error)"() -> (w322:errorcluster)
                      n160 = GPIB Write(0:w323, 1:"SS 1;", 2:3, 3:w322) -> (6:w321:errorcluster)  [unwired: 1 in, 1 out]
                      n161 = local write "error in (no error)"(w321) -> ()
                    }
                    frame #1 {
                      n162 = local read "error in (no error)"() -> (w327:errorcluster)
                      n163 = call "Time Delay13"("error in (no error)"=w327) -> ("error out"=w326:errorcluster)  [unwired: 10 in]
                      n164 = local write "error in (no error)"(w326) -> ()
                    }
                    frame #2 {
                      # "GPIB command to read the value of \nthe status byte, bit 1 Data Ready."
                      n165 = local read "error in (no error)"() -> (w328:errorcluster)
                      n166 = GPIB Read(0:w333, 1:10, 2:0, 3:w328) -> (5:w332:string, 7:w329:errorcluster)  [unwired: 1 in, 1 out]
                      n167 = local write "error in (no error)"(w329) -> ()
                      n168 = Decimal String To Number(string=w332) -> (number=w330:i32)  [unwired: 2 in, 1 out]
                      "Data Bit value" <- w330
                      n169 = Not Equal To 0?(x=w330) -> (x != 0?=w331:bool)
                    }
                    frame #3 {
                      n170 = local read "error in (no error)"() -> (w337:errorcluster)
                      n171 = call "Time Delay14"("error in (no error)"=w337) -> ("error out"=w336:errorcluster)  [unwired: 10 in]
                      n172 = local write "error in (no error)"(w336) -> ()
                    }
                  }
                }
              }
              frame #1 {
                # "Reads the scan position."
                n173 = local read "error in (no error)"() -> (w339:errorcluster)
                n174 = GPIB Write(0:w340, 1:"NN", 2:3, 3:w339) -> (6:w338:errorcluster)  [unwired: 1 in, 1 out]
                n175 = local write "error in (no error)"(w338) -> ()
              }
              frame #2 {
                n176 = local read "error in (no error)"() -> (w344:errorcluster)
                n177 = call "Time Delay20"("error in (no error)"=w344) -> ("error out"=w343:errorcluster)  [unwired: 10 in]
                n178 = local write "error in (no error)"(w343) -> ()
              }
              frame #3 {
                # "GPIB command to read the scan position."
                n179 = local read "error in (no error)"() -> (w346:errorcluster)
                n180 = GPIB Read(0:w349, 1:5, 2:3, 3:w346) -> (5:w348:string, 7:w345:errorcluster)  [unwired: 1 in, 1 out]
                n181 = local write "error in (no error)"(w345) -> ()
                n182 = Fract/Exp String To Number(string=w348) -> (number=w347:dbl)  [unwired: 3 in, 1 out]
                "# count periods done" <- w347
              }
              frame #4 {
                n183 = local read "error in (no error)"() -> (w353:errorcluster)
                n184 = call "Time Delay15"("error in (no error)"=w353) -> ("error out"=w352:errorcluster)  [unwired: 10 in]
                n185 = local write "error in (no error)"(w352) -> ()
              }
              frame #5 {
                # "Writes command to SR400\nto read the most recent complete\ndata point from counter A."
                n186 = local read "error in (no error)"() -> (w355:errorcluster)
                n187 = GPIB Write(0:w356, 1:"QA", 2:3, 3:w355) -> (6:w354:errorcluster)  [unwired: 1 in, 1 out]
                n188 = local write "error in (no error)"(w354) -> ()
              }
              frame #6 {
                n189 = local read "error in (no error)"() -> (w360:errorcluster)
                n190 = call "Time Delay18"("error in (no error)"=w360) -> ("error out"=w359:errorcluster)  [unwired: 10 in]
                n191 = local write "error in (no error)"(w359) -> ()
              }
              frame #7 {
                # "FOR loop reads the A counter \ndata buffer, converts string to\na number, writes into an array; \nas well, appends data into the path\ngiven filename \"a\".txt; finally, \nwrites to spreadsheet file."
                # "READ CHANNEL A DATA."
                # "Sends A counter data to\nthe default file."
                # "Sends A counter data to file '*a.txt'"
                n192 = local read "error in (no error)"() -> (w362:errorcluster)
                n193 = GPIB Read(0:w370, 1:20, 2:3, 3:w362) -> (5:w371:string, 7:w361:errorcluster)  [unwired: 1 in, 1 out]
                n194 = local write "error in (no error)"(w361) -> ()
                n195 = Fract/Exp String To Number(use system decimal point (T)=FALSE, string=w371) -> (number=w363:dbl)  [unwired: 2 in, 1 out]
                "counter A" <- w363
                n196 = Build Array(w366, w363) -> (w364:dbl[])
                n197 = Array To Spreadsheet String(array=w364, 3:"%e" ("format string")) -> (spreadsheet string=w367:string)  [unwired: 1 in]
                n198 = call <vilib>:"Write Characters To File.vi"("append to file? (new file:F)"=TRUE, "character string"=w367, "file path (dialog if empty)"=w365) -> ()  [unwired: 2 in, 1 out]
              }
              frame #8 {
                n199 = local read "error in (no error)"() -> (w376:errorcluster)
                n200 = call "Time Delay16"("error in (no error)"=w376) -> ("error out"=w375:errorcluster)  [unwired: 10 in]
                n201 = local write "error in (no error)"(w375) -> ()
              }
              frame #9 {
                # "Writes command to SR400\nto read the most recent complete\ndata point from counter B."
                n202 = local read "error in (no error)"() -> (w378:errorcluster)
                n203 = GPIB Write(0:w379, 1:"QB", 2:3, 3:w378) -> (6:w377:errorcluster)  [unwired: 1 in, 1 out]
                n204 = local write "error in (no error)"(w377) -> ()
              }
              frame #10 {
                n205 = local read "error in (no error)"() -> (w383:errorcluster)
                n206 = call "Time Delay17"("error in (no error)"=w383) -> ("error out"=w382:errorcluster)  [unwired: 10 in]
                n207 = local write "error in (no error)"(w382) -> ()
              }
              frame #11 {
                # "B counter data"
                # "count period #"
                # "B counter data read: Same \nprocedure as for the A counter.  \nAs well, for mode \nA for B, no data to read."
                # "READ CHANNEL B DATA."
                # "Sends B counter data to file '*b.txt'"
                n208 = local read "error in (no error)"() -> (w385:errorcluster)
                n209 = GPIB Read(0:w390, 1:20, 2:3, 3:w385) -> (5:w394:string, 7:w384:errorcluster)  [unwired: 1 in, 1 out]
                n210 = local write "error in (no error)"(w384) -> ()
                n211 = Fract/Exp String To Number(use system decimal point (T)=FALSE, string=w394) -> (number=w386:dbl)  [unwired: 2 in, 1 out]
                "counter B" <- w386
                n212 = Build Array(w389, w386) -> (w388:dbl[])
                n213 = Array To Spreadsheet String(array=w388, 3:"%e" ("format string")) -> (spreadsheet string=w391:string)  [unwired: 1 in]
                n214 = call <vilib>:"Write Characters To File.vi"("append to file? (new file:F)"=TRUE, "character string"=w391, "file path (dialog if empty)"=w387) -> ()  [unwired: 2 in, 1 out]
              }
              frame #12 {
                n215 = local read "error in (no error)"() -> (w399:errorcluster)
                n216 = call "Time Delay19"("error in (no error)"=w399) -> ("error out"=w398:errorcluster)  [unwired: 10 in]
                n217 = local write "error in (no error)"(w398) -> ()
              }
              frame #13 {
                # "Read Lockin Output"
                n218 = local read "Cluster"() -> (w407:T1)
                n219 = Unbundle By Name(w407) -> ("slope"=w406:i32, "Input Mode"=w405:i32, "time constant"=w404:i32, "display type"=w403:i32, "Range"=w402:i32)
                n220 = local read "error in (no error)"() -> (w401:errorcluster)
                n221 = call "SR5209 Read Output.vi"("VISA session (for class)"=w409, "Input Mode"=w405, "Time Constant"=w404, "Display Type"=w403, "Range"=w402, "error in (no error)"=w401, "Slope"=w406) -> ("Output (FP)"=w408:dbl, "error out"=w400:errorcluster)  [unwired: 4 in, 7 out]
                "lockin" <- w408
                n222 = local write "error in (no error)"(w400) -> ()
              }
              frame #14 {
                n223 = local read "error in (no error)"() -> (w411:errorcluster)
                n224 = call "Time Delay22"("error in (no error)"=w411) -> ("error out"=w410:errorcluster)  [unwired: 10 in]
                n225 = local write "error in (no error)"(w410) -> ()
              }
              frame #15 {
                # "lockin data"
                # "count period #"
                # "Sends lockin data to file '*c.txt'"
                n226 = Build Array(w413, w412) -> (w415:dbl[])
                n227 = Array To Spreadsheet String(array=w415, 3:"%e" ("format string")) -> (spreadsheet string=w416:string)  [unwired: 1 in]
                n228 = call <vilib>:"Write Characters To File.vi"("append to file? (new file:F)"=TRUE, "character string"=w416, "file path (dialog if empty)"=w414) -> ()  [unwired: 2 in, 1 out]
              }
              frame #16 {
                n229 = local read "error in (no error)"() -> (w420:errorcluster)
                n230 = call "Time Delay23"("error in (no error)"=w420) -> ("error out"=w419:errorcluster)  [unwired: 10 in]
                n231 = local write "error in (no error)"(w419) -> ()
              }
              frame #17 {
                # "lockin data"
                # "B counter data"
                # "A counter data"
                # "count period #"
                # "WRITE CHANNEL A, B DATA, and lockin data to default file."
                # "Sends count period #,\nA counter, B counter data,\nand lockin output \nto the default file."
                n232 = Build Array(w424, w426, w423, w422) -> (w425:dbl[])
                n233 = call-poly <vilib>:"Write To Spreadsheet File.vi"("transpose? (no:F)"=FALSE, "append to file? (new file:F)"=TRUE, "1D data"=w425, "file path (dialog if empty)"=w421) -> ()  [unwired: 4 in, 1 out]
              }
              frame #18 {
                n234 = local read "error in (no error)"() -> (w430:errorcluster)
                n235 = call "Time Delay21"("error in (no error)"=w430) -> ("error out"=w429:errorcluster)  [unwired: 10 in]
                n236 = local write "error in (no error)"(w429) -> ()
              }
              frame #19 {
                # "Counter B graph"
                # "Counter A graph"
                n237 = call-poly <vilib>:"Read From Spreadsheet File.vi"("format (%.3f)"="%e", "file path (dialog if empty)"=w445) -> ("all rows"=w435:dbl[][])  [unwired: 5 in, 4 out]
                n238 = call-poly <vilib>:"Read From Spreadsheet File.vi"("format (%.3f)"="%e", "file path (dialog if empty)"=w432) -> ("all rows"=w440:dbl[][])  [unwired: 5 in, 4 out]
                n239 = Delete From Array(array=w435, index (col)=0 ("disabled index (col)")) -> (deleted portion=w436:dbl[])  [unwired: 2 in, 1 out]
                n240 = Delete From Array(array=w435, index (col)=1 ("disabled index (col)")) -> (deleted portion=w437:dbl[])  [unwired: 2 in, 1 out]
                n241 = Delete From Array(array=w440, index (col)=0 ("disabled index (col)")) -> (deleted portion=w442:dbl[])  [unwired: 2 in, 1 out]
                n242 = Delete From Array(array=w440, index (col)=1 ("disabled index (col)")) -> (deleted portion=w441:dbl[])  [unwired: 2 in, 1 out]
                n243 = Bundle "Bundle"("all rows"=w436, "all rows"=w437) -> (w433:cluster{"all rows":dbl[], "all rows":dbl[]})  [unwired: 1 in]
                n244 = Bundle "Bundle"("all rows"=w442, "all rows"=w441) -> (w434:cluster{"all rows":dbl[], "all rows":dbl[]})  [unwired: 1 in]
                n245 = Build Array(w434, w433) -> (→"PHOTON COUNTER DATA":cluster{"all rows":dbl[], "all rows":dbl[]}[])
              }
              frame #20 {
                # "Send to Graph"
                # "Lockin graph"
                n246 = call-poly <vilib>:"Read From Spreadsheet File.vi"("format (%.3f)"="%e", "file path (dialog if empty)"=w448) -> ("all rows"=w455:dbl[][])  [unwired: 5 in, 4 out]
                n247 = Delete From Array(array=w455, index (col)=0 ("disabled index (col)")) -> (deleted portion=w450:dbl[])  [unwired: 2 in, 1 out]
                n248 = Delete From Array(array=w455, index (col)=1 ("disabled index (col)")) -> (deleted portion=w449:dbl[])  [unwired: 2 in, 1 out]
                n249 = call "Convert to Dynamic Data"("Array"=w450) -> ("Dynamic Data Type"=w452:dynamicdata)  [unwired: 3 in]
                n250 = call "Convert to Dynamic Data2"("Array"=w449) -> ("Dynamic Data Type"=w451:dynamicdata)  [unwired: 3 in]
                n251 = call "Build XY Graph"("Y Input"=w451, "X Input"=w452) -> ("XY Graph"=→"LOCKIN OUTPUT DATA":cluster{"Y":dbl[], "Y":dbl[]}[])  [unwired: 8 in, 1 out]
              }
            }
          }
        }
        frame #3 {
          # "CLEAR STATUS BYTE, SEND STATUS."
          n252 = local read "error in (no error)"() -> (w459:errorcluster)
          n253 = GPIB Write(0:w460, 1:"SS", 2:3, 3:w459) -> (6:w458:errorcluster)  [unwired: 1 in, 1 out]
          n254 = local write "error in (no error)"(w458) -> ()
        }
        frame #4 {
          # "CLEAR STATUS."
          n255 = local read "error in (no error)"() -> (w464:errorcluster)
          n256 = GPIB Read(0:w465, 1:6, 2:0, 3:w464) -> (7:w463:errorcluster)  [unwired: 1 in, 2 out]
          n257 = local write "error in (no error)"(w463) -> ()
        }
      }
    }
    frame #27 {
      # "Save the data to a file and location\nspecified by the user."
      n258 = Two Button Dialog(message="Would you like to save the graph?", 1:"Don't Save" ("F button name (\"Cancel\")"), 2:"Save" ("T button name (\"OK\")")) -> (T button?=w468:bool)
      n259 = case shown="True" w468 {
        tunnel: w469 -> [_ w473]
        frame False {
        }
        frame True {
          n260 = stacked-sequence {
            seq-local: [w475 _] -> [_ w477]
            tunnel: w473 -> [w474 _]
            frame #0 {
              n261 = call-poly <vilib>:"Read From Spreadsheet File.vi"("format (%.3f)"="%e", "file path (dialog if empty)"=w474) -> ("all rows"=w475:dbl[][])  [unwired: 5 in, 4 out]
            }
            frame #1 {
              n262 = call-poly <vilib>:"Write To Spreadsheet File.vi"("format (%.3f)"="%e", "2D data"=w477) -> ()  [unwired: 6 in, 1 out]
            }
          }
        }
      }
    }
  }
  n263 = local write "Cluster"("Cluster") -> ()
  n264 = local write "error in (no error)"("error in (no error)") -> ()
